vi "GetCustomData.vi"(8 "error in":errorcluster, 11 "ProductUnit in":refnum<class "ProductUnit.lvclass">) -> (0 "error out":errorcluster, 2 "CustomData":refnum<class "CustomData.lvclass">, 3 "ProductUnit out":refnum<class "ProductUnit.lvclass">)   [LabVIEW 2021, in "ProligentXMLGenerator.lvlib" / "ProductUnit.lvclass"]
doc: "Get CustomData\n\nThe values defined under this element will not be interpreted by the DIT. It can be used to store data that will be used by another system."
uses:
  ProductUnit.lvclass
  ProductUnit.lvclass/ProductUnit.ctl
  Model/CustomData/CustomData.lvclass
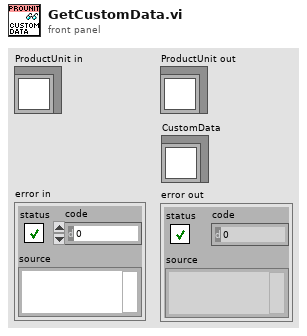
[diagram p1: front panel]
types:
  T1 = typedef "ProligentXMLGenerator.lvlib/ProductUnit.lvclass/Data.ctl" = cluster{"Name":string, "Characteristics":refnum<class "Characteristic.lvclass">[], "Documents":refnum<class "Document.lvclass">[], "CustomData":refnum<class "CustomData.lvclass">, "ProductUnitIdentifier":refnum<class "NonEmptyString_50.lvclass">, "ProductFullName":refnum<class "FullName.lvclass">, "Scrapped":refnum<class "Boolean.lvclass">, "ScrappedTime":refnum<class "DateTime.lvclass">, "CreationTime":refnum<class "DateTime.lvclass">, "ManufacturingTime":refnum<class "DateTime.lvclass">, "ByManufacturer":refnum<class "NonEmptyString_255.lvclass">, "TimeZoneInfoId":string}
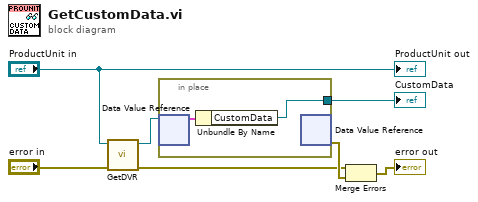
[diagram p0: block diagram]
diagram:
  n1 = call "GetDVR.vi"("error in"="error in", "ProductUnit in"="ProductUnit in") -> ("error out"=w1:errorcluster, "DVRReference"=w6:refnum<data-value>)  [unwired: 8 in]
  n2 = in-place "In Place Element Structure" {
    in-place-border: [w8] -> w2
    n3 = in-place-dvr #1(w6) -> (w9:T1)  [unwired: 1 out]
    n4 = Unbundle By Name(w9) -> ("CustomData"=w8:refnum<class "CustomData.lvclass">)
    n5 = in-place-dvr #1() -> (w7:errorcluster)  [unwired: 1 in, 1 out]
  }
  "CustomData" <- w2
  n6 = Merge Errors(w1, w7) -> (→"error out":errorcluster)
  "ProductUnit out" <- "ProductUnit in"
